vi "Get Plot ID.vi"(8 "error in (no error)":errorcluster, 11 "3D Contour Datatype.lvclass in":refnum<class "3D Contour Datatype.lvclass">) -> (0 "error out":errorcluster, 1 "Plot ID":i32, 3 "3D Contour Datatype.lvclass out":refnum<class "3D Contour Datatype.lvclass">)   [LabVIEW 2020, in "3D Contour Datatype.lvclass"]
uses:
  <vilib>/Math Plots/3D Math Plots/3D Contour/3D Contour Datatype/3D Contour Datatype.lvclass
  <vilib>/Math Plots/3D Math Plots/3D Contour/3D Contour Datatype/3D Contour Datatype.lvclass/3D Contour Datatype.ctl
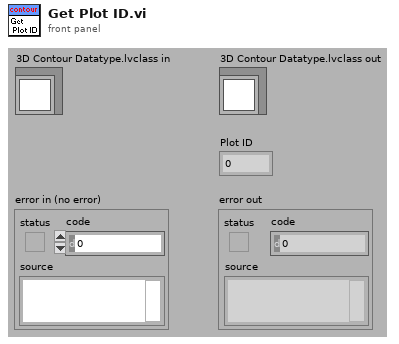
[diagram p1: front panel]
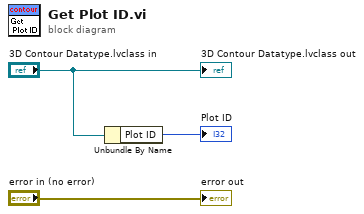
[diagram p0: block diagram]
diagram:
  n1 = Unbundle By Name("3D Contour Datatype.lvclass in") -> ("Plot ID"=→"Plot ID":i32)
  "3D Contour Datatype.lvclass out" <- "3D Contour Datatype.lvclass in"
  "error out" <- "error in (no error)"
